vi "Message State Machine.vi"(8 "error in (no error)":errorcluster, 11 "Message":string) -> (0 "error out":errorcluster)   [LabVIEW 2019]
uses:
  Typedefs/Message States.ctl
  Typedefs/Sensor Types.ctl
  Typedefs/Message Types.ctl
  Typedefs/Message.ctl
  Comms/State Controller/Controls/Comms Loop States.ctl
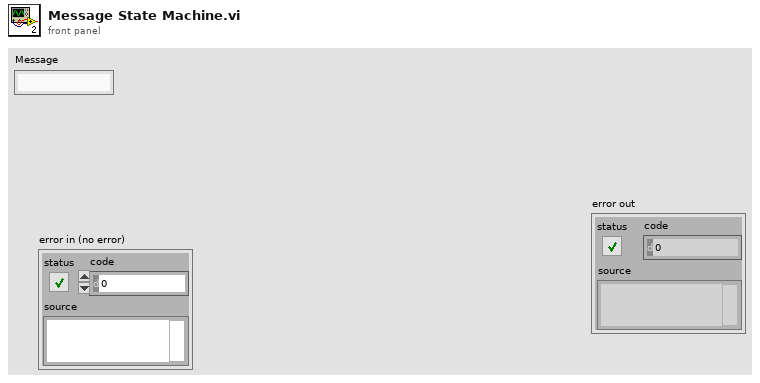
[diagram p1: front panel]
types:
  T1 = typedef "Message States.ctl" = enum16{"START", "PAYLOAD", "SEQUENCE", "SENSOR_TYPE", "MESSAGE_ID", "DATA"}
  T2 = typedef "Message.ctl" = cluster{"Payload Size":u8, "Sequence Number":u8, "Sensor Type":T3, "Message Types":T4, "Data":u8[]}
  T3 = typedef "Sensor Types.ctl" = enum16{"APP", "TURBIDITY", "PH"}
  T4 = typedef "Message Types.ctl" = enum16{"HEART_BEAT", "CONNECT", "GET_CURRENT_MEASUREMENTS", "GET_LOG_FILE", "SEND_LOG_FILE_SIZE", "SEND_LOG_FILE_CHUNK", "GET_LOGGING_PERIOD", "SET_LOGGING_PERIOD", "SEND_SD_CARD_INFO", "GET_LOGS_LIST", "SEND_LOG_FILE_NAME", "SEND_LOGGING_PERIOD", "GET_RTC_TIME", "SET_RTC_TIME", "SEND_RTC_TIME", "SEND_CURRENT_MEASUREMENTS", "DELETE_LOG_FILE", "GET_SD_CARD_INFO", "GET_BATTERY_INFO", "SEND_BATTERY_INFO", "GET_LOG_FILE_SIZE", "ERROR_MSG"}
  T5 = typedef "Comms Loop States.ctl" = enum16{"Initalise", "User Event", "Parse New Message", "SEND_LOG_FILE_NAME"}
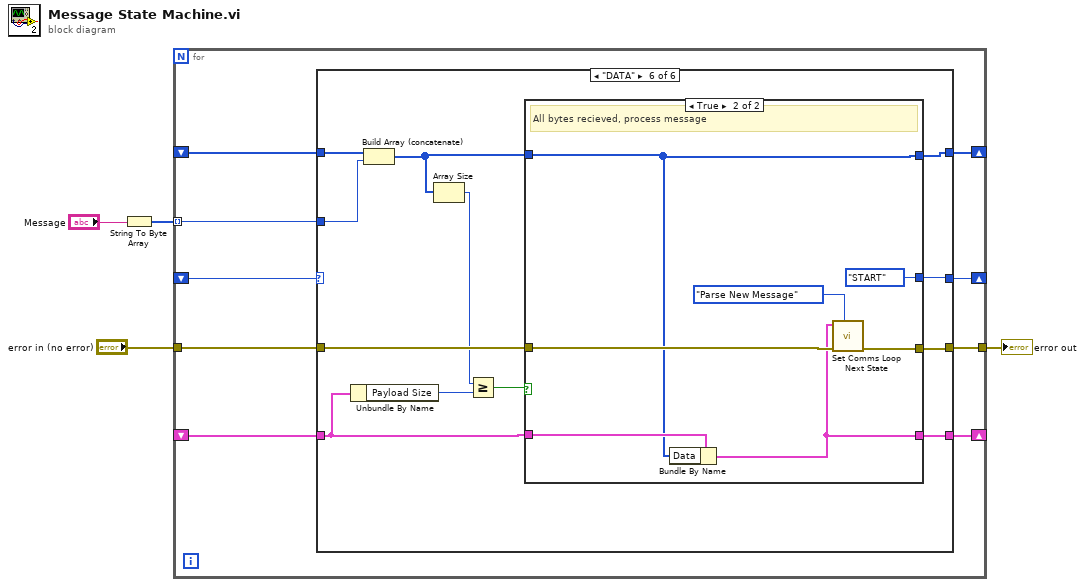
[diagram p0: block diagram]
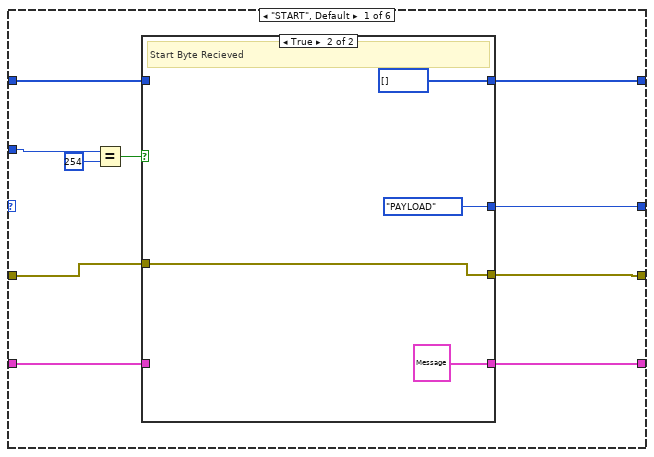
[diagram p2: hidden frame]
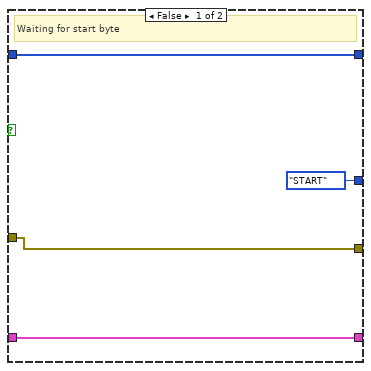
[diagram p3: hidden frame]
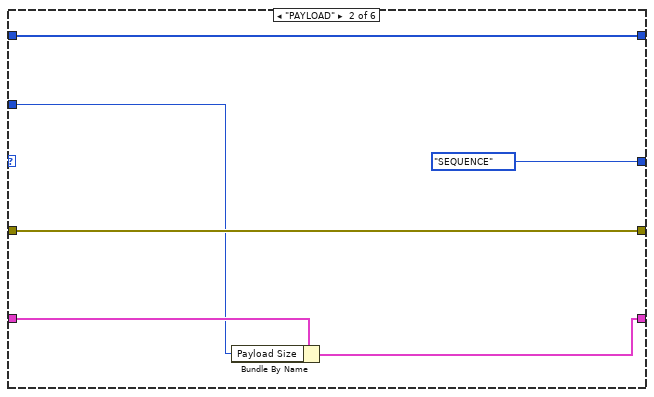
[diagram p4: hidden frame]
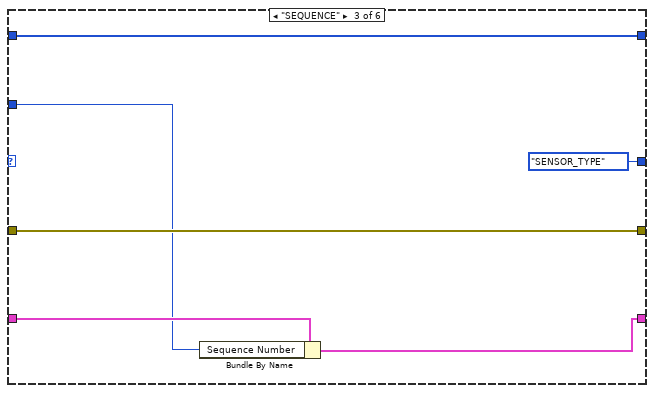
[diagram p5: hidden frame]
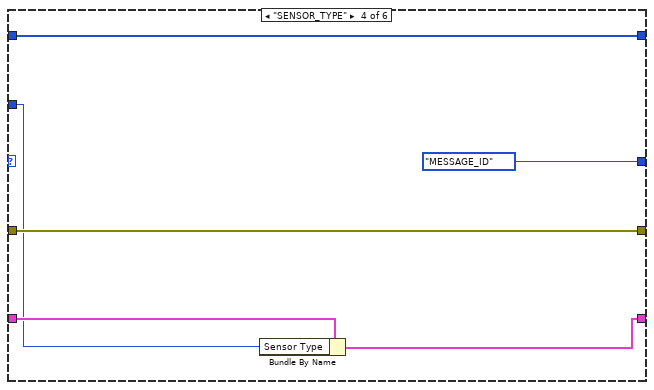
[diagram p6: hidden frame]
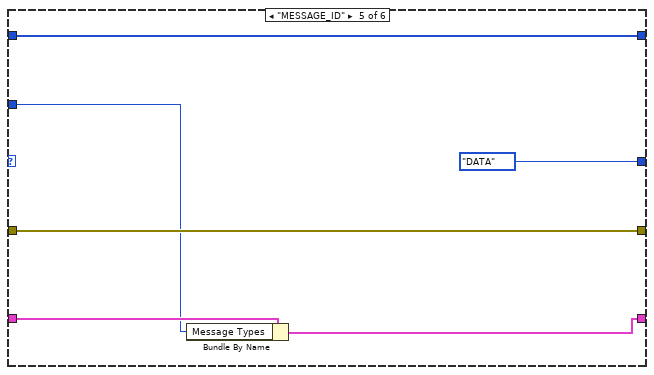
[diagram p7: hidden frame]
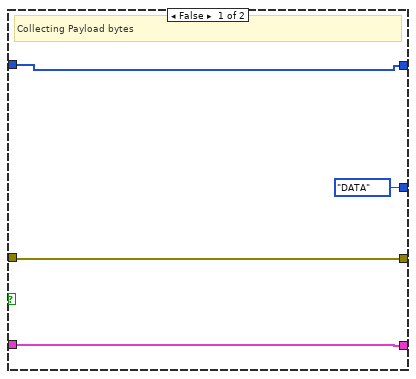
[diagram p8: hidden frame]
diagram:
  n1 = String To Byte Array(string="Message") -> (unsigned byte array=w1:u8[])
  n2 = for {
    shift-right: [w7] -> _
    shift-left: _ -> [w13]
    tunnel: "error in (no error)" -> [w12]
    tunnel: [w11] -> w3
    tunnel: w1 -> [w10] mode=indexing
    shift-right: [w8] -> _
    shift-left: _ -> [w9]
    shift-right: [w6] -> _
    shift-left: _ -> [w5]
    n3 = case shown="\"DATA\"" w13 {
      tunnel: w12 -> [w17 w37 w43 w49 w55 w64]
      tunnel: [w18 w37 w43 w49 w55 w62] -> w11
      tunnel: w10 -> [w23 w33 w41 w45 w51 w57]
      tunnel: w9 -> [w16 w36 w38 w48 w53 w59]
      tunnel: [w20 w36 w38 w48 w53 w60] -> w8
      tunnel: [w19 Message_States."SEQUENCE" ("Message State Machine State") Message_States."SENSOR_TYPE" ("Message State Machine State") Message_States."MESSAGE_ID" ("Message State Machine State") Message_States."DATA" ("Message State Machine State") w61] -> w7
      tunnel: [w15 w32 w40 w44 w50 w63] -> w6
      tunnel: w5 -> [w14 w34 w42 w46 w52 w65]
      frame "START", Default {
        n4 = Equal?(x=w23, y=u8 254) -> (x = y?=w21:bool)
        n5 = case shown="True" w21 {
          tunnel: [w27 u8[] []] -> w20
          tunnel: [Message_States."START" ("Message State Machine State") Message_States."PAYLOAD" ("Message State Machine State")] -> w19
          tunnel: [w25 w29] -> w18
          tunnel: w17 -> [w25 w29]
          tunnel: w16 -> [w27 _]
          tunnel: [w24 T2 {"Payload Size"=0, "Sequence Number"=0, "Sensor Type"=enum."APP", "Message Types"=enum."SEND_LOG_FILE_SIZE", "Data"=[]} ("Message")] -> w15
          tunnel: w14 -> [w24 _]
          frame False {
            # "Waiting for start byte"
          }
          frame True {
            # "Start Byte Recieved"
          }
        }
      }
      frame "PAYLOAD" {
        n6 = Bundle By Name(cluster=w34, "Payload Size"=w33) -> (w32:T2)
      }
      frame "SEQUENCE" {
        n7 = Bundle By Name(cluster=w42, "Sequence Number"=w41) -> (w40:T2)
      }
      frame "SENSOR_TYPE" {
        n8 = Bundle By Name(cluster=w46, "Sensor Type"=w45) -> (w44:T2)
      }
      frame "MESSAGE_ID" {
        n9 = Bundle By Name(cluster=w52, "Message Types"=w51) -> (w50:T2)
      }
      frame "DATA" {
        n10 = Unbundle By Name(w65) -> ("Payload Size"=w67:u8)
        n11 = Build Array (concatenate)(w59, w57) -> (w58:u8[])
        n12 = Array Size(array=w58) -> (size(s)=w56:i32)
        n13 = Greater Or Equal?(x=w56, y=w67) -> (x >= y?=w66:bool)
        n14 = case shown="True" w66 {
          tunnel: w65 -> [w71 w78]
          tunnel: w58 -> [w70 w72]
          tunnel: w64 -> [w68 w77]
          tunnel: [w71 w76] -> w63
          tunnel: [w68 w74] -> w62
          tunnel: [Message_States."DATA" ("Message State Machine State") Message_States."START" ("Message State Machine State")] -> w61
          tunnel: [w70 w72] -> w60
          frame False {
            # "Collecting Payload bytes"
          }
          frame True {
            # "All bytes recieved, process message"
            n15 = Bundle By Name(cluster=w78, "Data"=w72) -> (w76:T2)
            n16 = call "Set Comms Loop Next State.vi"("Command"=Comms_Loop_States."Parse New Message", "error in (no error)"=w77, "Data"=w76) -> ("error out"=w74:errorcluster)  [unwired: 8 in]
          }
        }
      }
    }
  }
  "error out" <- w3
